vi "Locate Sensor.vi"() -> ()   [LabVIEW 2016]
uses:
  Drivers/Aerotech A3200/Aerotech VIs.lvlib
panel:
  in  "Joystick":bool=TRUE
  out "Calibrated Results (Top Left, Bottom Right)":sgl[][](array[numeric]) format="%.2f"
  in  "Vision Type":T1(ring)
  in  "Stop":bool
  out "Image Out":T2(plugin-control)
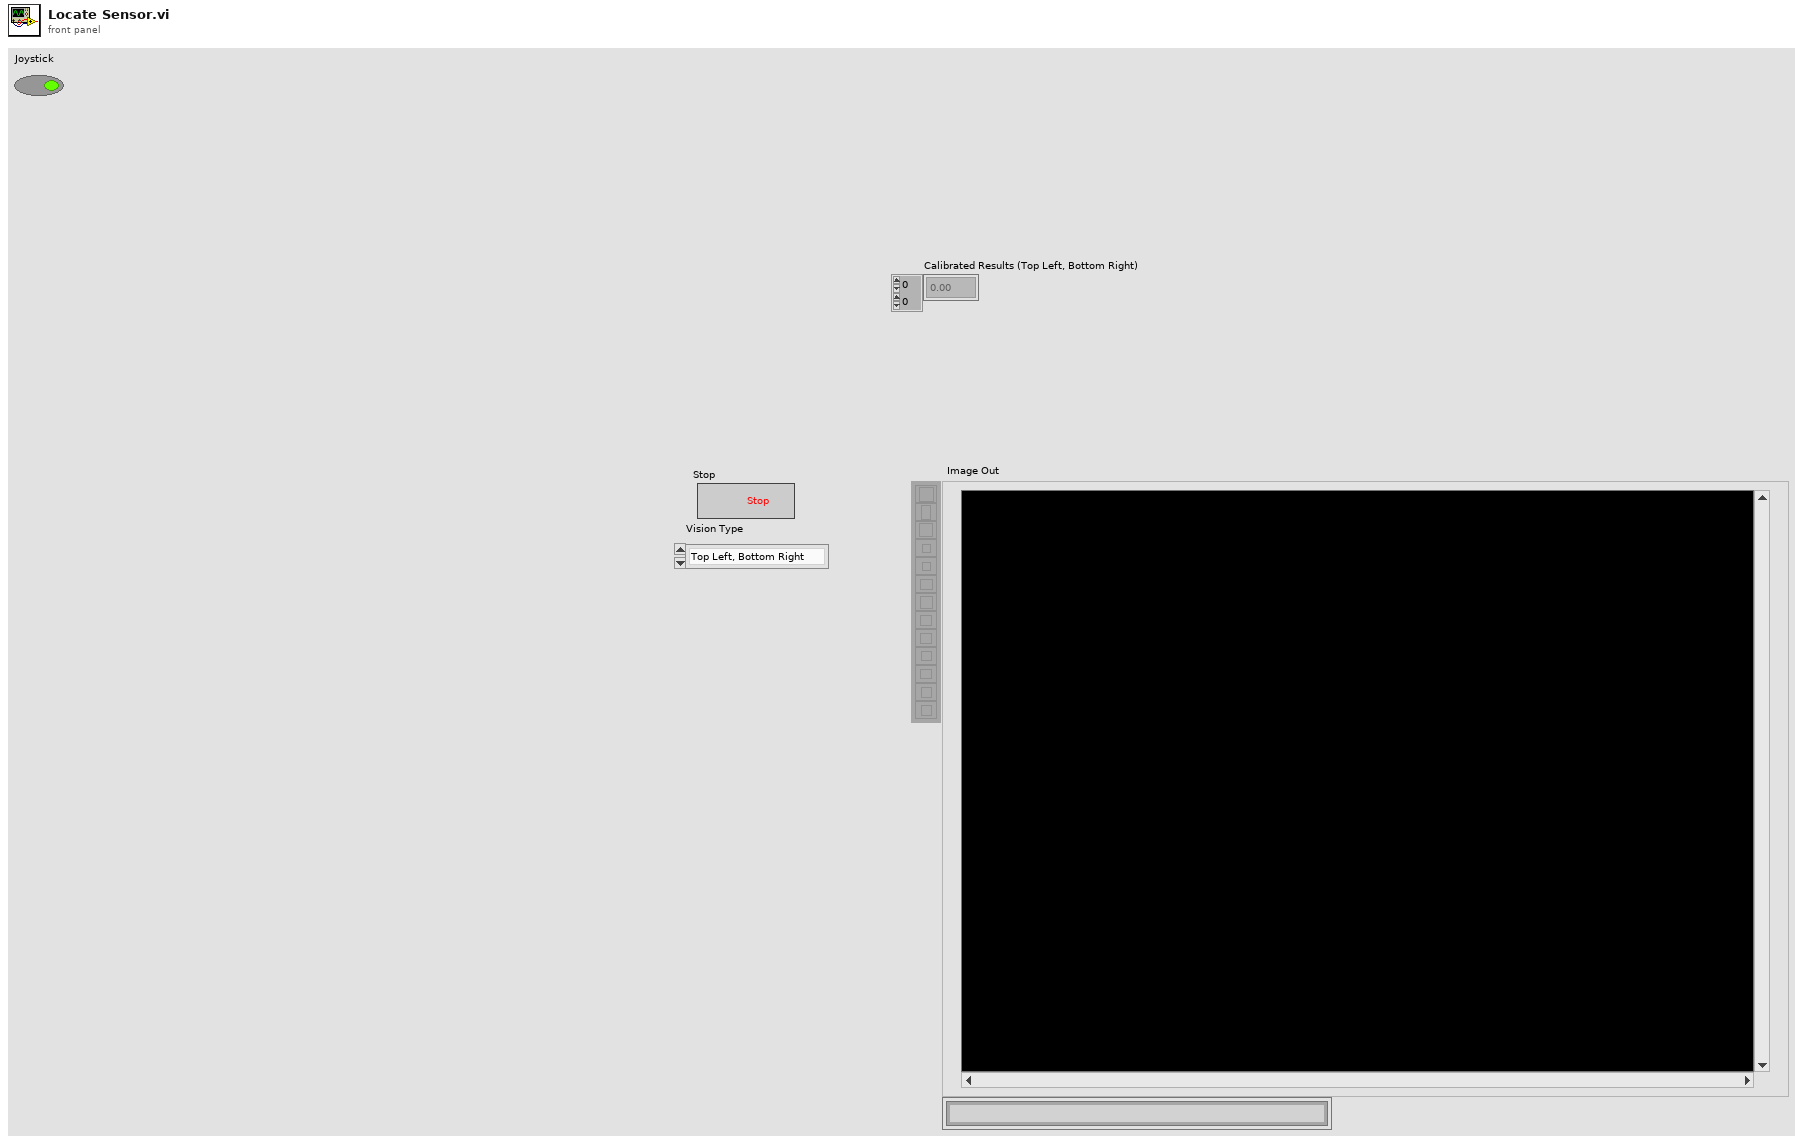
[diagram p1: front panel]
types:
  T1 = enum16{"Top Left, Bottom Right", "Bottom Left, Top Right"}
  T2 = typedef "IMAQ Image.ctl" = refnum<image>
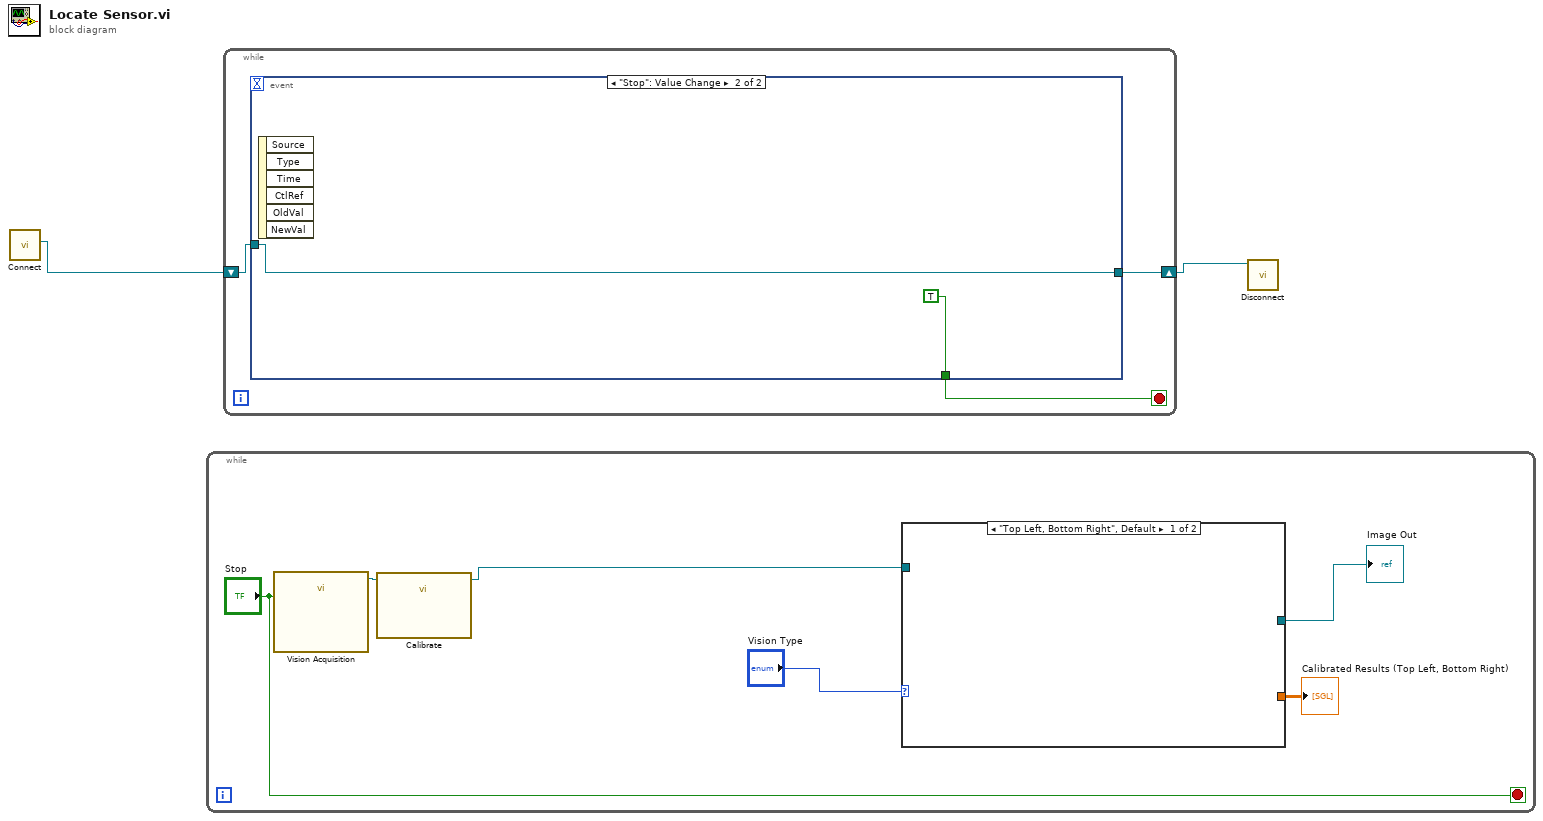
[diagram p0: block diagram]
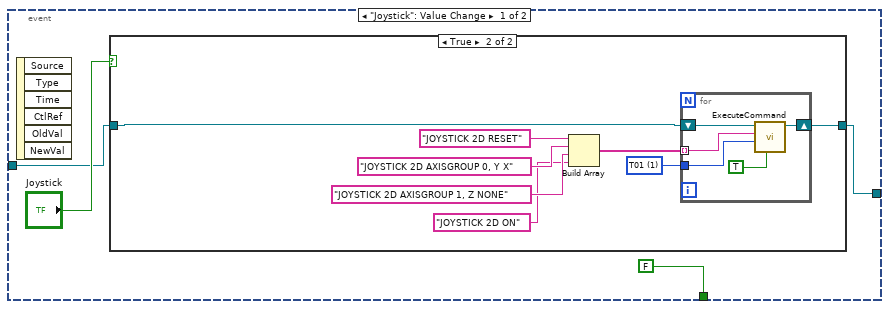
[diagram p2: hidden frame]
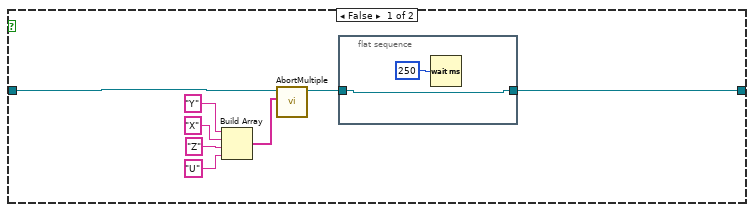
[diagram p3: hidden frame]
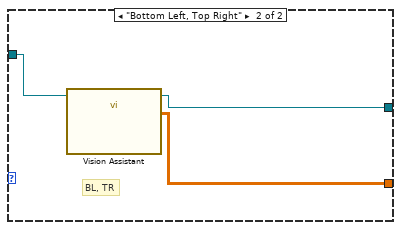
[diagram p4: hidden frame]
diagram:
  n1 = call "Connect.vi"() -> ("controller"=w2:refnum<k24>)  [unwired: 10 in, 1 out]
  n2 = while {
    stop <- "Stop" stop-if-true
    n3 = call "Vision Acquisition"("Stop (F)"="Stop") -> ("Image Out"=w8:T2)  [unwired: 24 in, 2 out]
    n4 = call "Calibrate"("Image In"=w8) -> ("Image Out"=w6:T2)  [unwired: 25 in, 1 out]
    n5 = case shown="\"Top Left, Bottom Right\", Default" "Vision Type" {
      tunnel: w6 -> [_ w11]
      tunnel: [_ w10] -> w5
      tunnel: [_ w9] -> w4
      frame "Top Left, Bottom Right", Default {
      }
      frame "Bottom Left, Top Right" {
        # "BL, TR"
        n6 = call "Vision Assistant"("Image In"=w11) -> ("Image Out"=w10:T2, "Calibrated Results (Bottom Left, Top Right)"=w9:sgl[][])  [unwired: 23 in, 2 out]
      }
    }
    "Image Out" <- w5
    "Calibrated Results (Top Left, Bottom Right)" <- w4
  }
  n7 = while {
    shift-right: [w13] -> w1
    shift-left: w2 -> [w14]
    stop <- w12 stop-if-true
    n8 = event shown="[1] \"Stop\": Value Change" {
      selector: _ -> [_ _]
      dyn-events: _ -> [_ _]
      timeout: _ -> [_ _]
      tunnel: w14 -> [w17 w42]
      tunnel: [w16 w42] -> w13
      tunnel: [FALSE TRUE] -> w12
      event "Joystick": Value Change {
        n9 = event-data() -> ()  [unwired: 1 in, 6 out]
        n10 = case shown="True" "Joystick" {
          tunnel: w17 -> [w20 w30]
          tunnel: [w19 w29] -> w16
          frame False {
            n11 = Build Array("Y" ("axis name"), "X", "Z", "U") -> (w22:string[])
            n12 = call "AbortMultiple.vi"("axis names"=w22, "controller in"=w20) -> ("controller out"=w21:refnum<k24>)  [unwired: 8 in, 1 out]
            n13 = flat-sequence {
              tunnel: w21 -> [w28]
              tunnel: [w28] -> w19
              frame #0 {
                n14 = Wait (ms)(milliseconds to wait=u32 250) -> ()  [unwired: 1 out]
              }
            }
          }
          frame True {
            w32 = 1 items=["TLibrary", "T01", "T02", "T03", "T04", "T05", "T06", "T07", "T08", "T09", "T10", "T11", "T12", "T13", "T14", "T15", "T16", "T17", "T18", "T19", "T20", "T21", "T22", "T23", "T24", "T25", "T26", "T27", "T28", "T29", "T30", "T31"] ("taskId")
            n15 = Build Array("JOYSTICK 2D RESET", "JOYSTICK 2D AXISGROUP 0, Y X", "JOYSTICK 2D AXISGROUP 1, Z NONE", "JOYSTICK 2D ON") -> (w33:string[])
            n16 = for {
              tunnel: w33 -> [w41] mode=indexing
              tunnel: w32 -> [w40]
              shift-right: [w37] -> w29
              shift-left: w30 -> [w39]
              n17 = call "ExecuteCommand.vi"("return immediately"=TRUE, "taskId"=w40, "Command Code"=w41, "controller in"=w39) -> ("controller out"=w37:refnum<k24>)  [unwired: 5 in, 2 out]
            }
          }
        }
      }
      event "Stop": Value Change {
        n18 = event-data() -> ()  [unwired: 1 in, 6 out]
      }
    }
  }
  n19 = call "Disconnect.vi"("controller"=w1) -> ()  [unwired: 10 in, 1 out]
